vi "Diff View.vi"(10 "Diffed Text":string) -> ()   [LabVIEW 2020, in "Approval Tests.lvlib" / "Report With Native Compare Tool.lvclass"]
uses:
  Report With Native Compare Tool.lvclass
  astemes-string-diff-utils/source/Find Highlights.vi
panel:
  out "Diff View":string
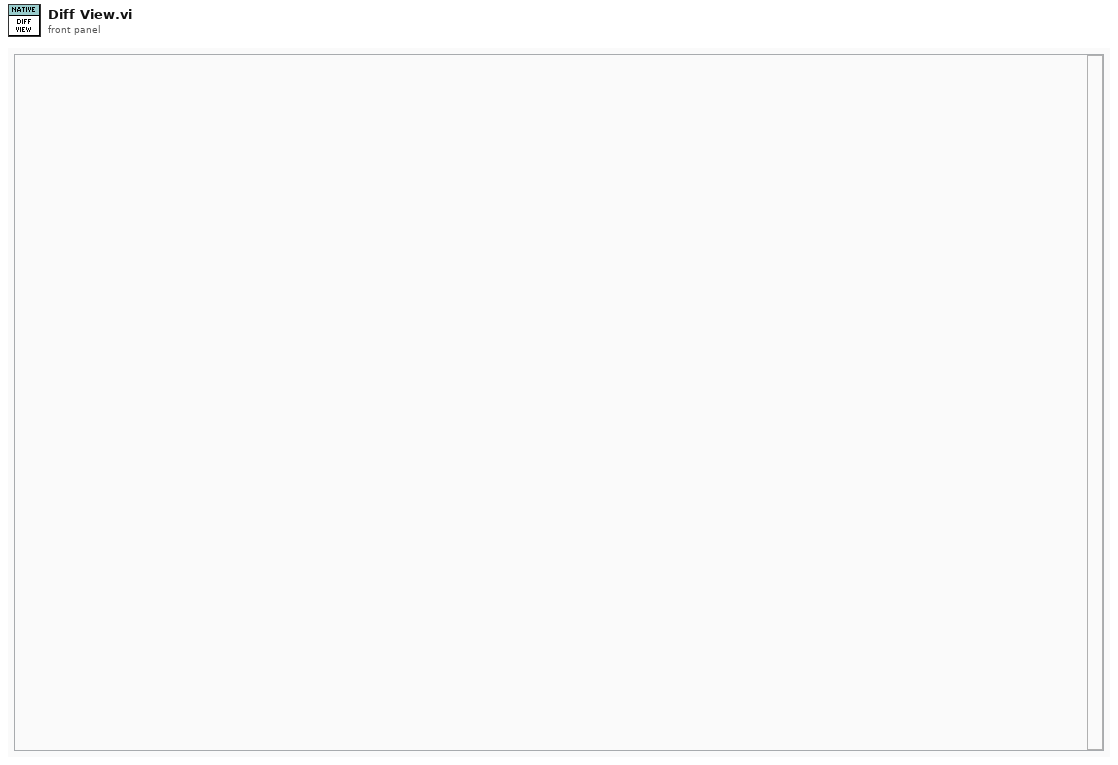
[diagram p1: front panel]
types:
  T1 = cluster{"Selection Start":u32, "Selection End":u32, "Type":enum16{"added", "missing"}}[]
  T2 = cluster{"Text.Selection":cluster{"Selection Start":u32, "Selection End":u32}, "Color":u32}
  T3 = cluster{"Selection Start":u32, "Selection End":u32}
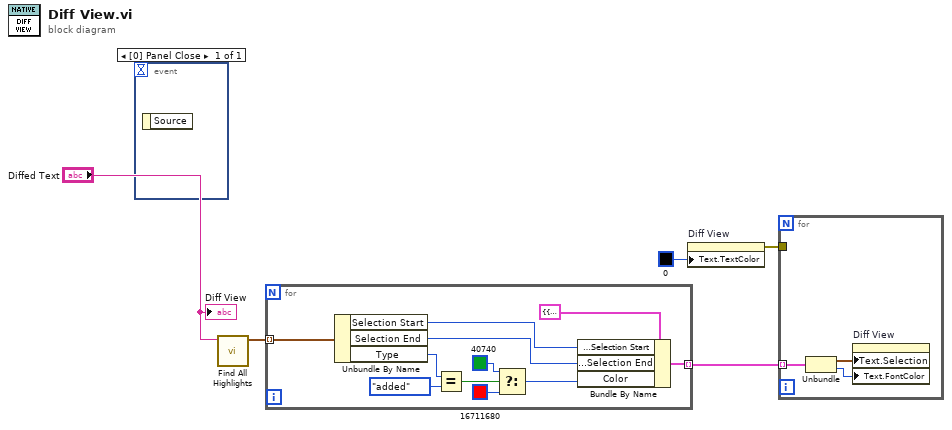
[diagram p0: block diagram]
diagram:
  n1 = event shown="[0] Panel Close" {
    selector: _ -> [_]
    dyn-events: _ -> [_]
    timeout: _ -> [_]
    event Panel Close {
      n2 = event-data() -> ()  [unwired: 1 in, 1 out]
    }
  }
  n3 = call "Find All Highlights.vi"("String"="Diffed Text") -> ("Sections"=w2:T1)  [unwired: 10 in]
  n4 = for {
    tunnel: w2 -> [w16] mode=indexing
    tunnel: [w10] -> w4 mode=indexing
    n5 = Unbundle By Name(w16) -> ("Selection Start"=w14:u32, "Selection End"=w13:u32, "Type"=w12:enum16{"added", "missing"})
    n6 = Equal?(x=w12, y=enum16{"added", "missing"}."added") -> (x = y?=w9:bool)
    n7 = Select(t=u32 40740 ("Text.Text Colors:Text Color"), s=w9, f=u32 16711680 ("Text.Text Colors:Text Color")) -> (s? t:f=w6:u32)
    n8 = Bundle By Name(cluster=T2 {"Text.Selection"={"Selection Start"=0, "Selection End"=0}, "Color"=40740} ("Colors"), "Text.Selection.Selection Start"=w14, "Text.Selection.Selection End"=w13, "Color"=w6) -> (w10:T2)
  }
  n9 = property on="Diff View" class="Str"("Text.TextColor"=u32 0 ("Text.Text Colors:Text Color")) -> (error out=w5:errorcluster)  [unwired: 2 in, 1 out]
  n10 = for {
    tunnel: w4 -> [w17] mode=indexing
    tunnel: w5 -> [_]
    n11 = Unbundle(w17) -> ("Text.Selection"=w19:T3, "Color"=w18:u32)
    n12 = property on="Diff View" class="Str"("Text.Selection"=w19, "Text.FontColor"=w18) -> ()  [unwired: 2 in, 2 out]
  }
  "Diff View" <- "Diffed Text"
